vi "Ask Permission.vi"(7 "scope":string="read_station", 8 "error in (no error)":errorcluster, 9 "client id":string="581786658708-elflankerquo1a6vsckabbhn25hclla0.apps.googleusercontent.com", 10 "redirect uri":string="http://127.0.0.1:8001/oAuth/Redirect", 11 "authorization endpoint":string="https://api.netatmo.com/oauth2/authorize") -> (0 "error out":errorcluster, 3 "original state":string)   [LabVIEW 2020, in "Netatmo-WeatherStation.lvlib"]
uses:
  Netatmo-WeatherStation.lvlib
panel:
  out "full URL":string
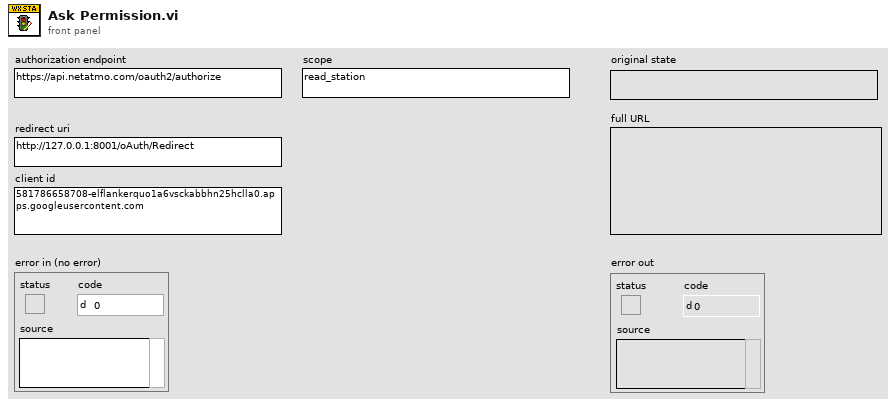
[diagram p1: front panel]
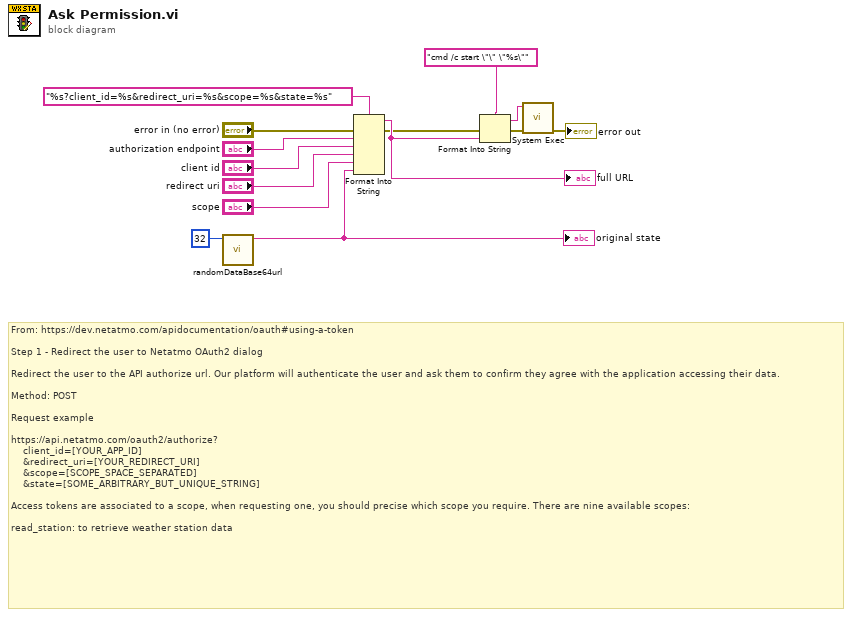
[diagram p0: block diagram]
diagram:
  # "From: https://dev.netatmo.com/apidocumentation/oauth#using-a-token\n\nStep 1 - Redirect the user to Netatmo OAuth2 dialog\n\nRedirect the user to the API authorize url. Our platform will authenticate the user and ask them to confirm they agree with the application accessing their data.\n\nMethod: POST\n\nRequest example\n\nhttps://api.netatmo.com/oauth2/authorize?\n    client_id=[YOUR_APP_ID]\n    &redirect_uri=[YOUR_REDIRECT_URI]\n    &scope=[SCOPE_SPACE_SEPARATED]\n    &state=[SOME_ARBITRARY_BUT_UNIQUE_STRING]\n\nAccess tokens are associated to a scope, when requesting one, you should precise which scope you require. There are nine available scopes:\n\nread_station: to retrieve weather station data"
  n1 = call "randomDataBase64url.vi"("length"=32) -> ("base64 string"=w3:string)  [unwired: 10 in]
  "original state" <- w3
  n2 = Format Into String(format string="%s?client_id=%s&redirect_uri=%s&scope=%s&state=%s" ("command line"), error in="error in (no error)", "authorization endpoint", "client id", "redirect uri", "scope", w3) -> (resulting string=w11:string, error out=w8:errorcluster)  [unwired: 1 in]
  "full URL" <- w11
  n3 = Format Into String(format string="cmd /c start \"\" \"%s\"" ("command line"), error in=w8, w11) -> (resulting string=w14:string, error out=w6:errorcluster)  [unwired: 1 in]
  n4 = call <vilib>:"System Exec.vi"("error in (no error)"=w6, "command line"=w14) -> ("error out"=→"error out":errorcluster)  [unwired: 6 in, 3 out]
